vi "Weighted Checksum.vi"(10 "Weight":u32, 11 "Text":string) -> (3 "Checksum":u32)   [LabVIEW 2019, in "Instrument.Lockin.lvlib" / "Instrument.Lockin.lvclass"]
uses:
  Instrument.Lockin.lvclass
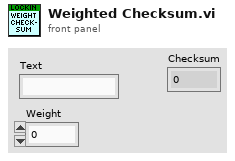
[diagram p1: front panel]
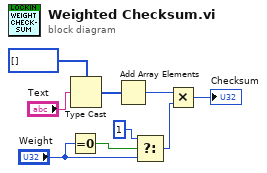
[diagram p0: block diagram]
diagram:
  n1 = Equal To 0?(x="Weight") -> (x = 0?=w5:bool)
  n2 = Type Cast(type=u32[] [], x="Text") -> (*(type *) &x=w7:u32[])
  n3 = Add Array Elements(numeric array=w7) -> (sum=w8:u32)
  n4 = Select(t=u32 1, s=w5, f="Weight") -> (s? t:f=w3:u32)
  n5 = Multiply(x=w8, y=w3) -> (x*y=→"Checksum":u32)
